vi "Raw Data.vi"(0 "reference in":refnum<class "Advantech.lvclass">, 5 "error in (no error)":errorcluster) -> (14 "reference out":refnum<class "Advantech.lvclass">, 15 "Raw Data":dbl, 19 "error out":errorcluster)   [LabVIEW 2013, in "Advantech.lvclass"]
uses:
  Advantech.lvclass
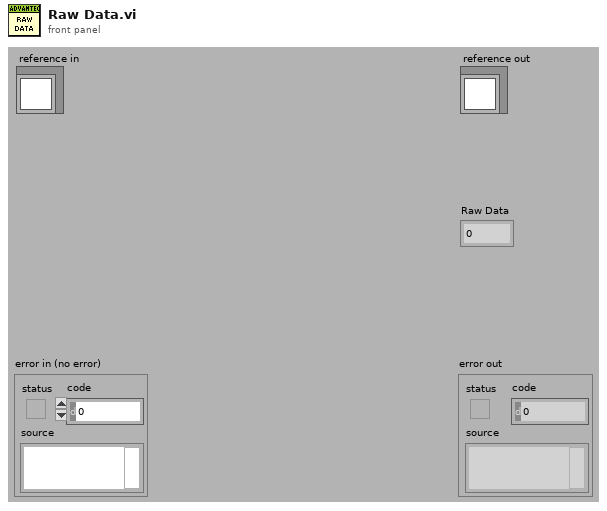
[diagram p1: front panel]
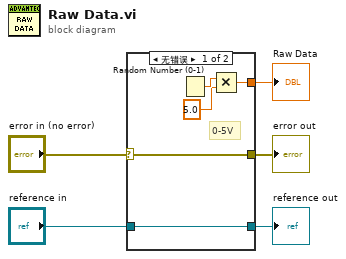
[diagram p0: block diagram]
diagram:
  n1 = case shown="无错误" "error in (no error)" {
    selector: "error in (no error)" -> [w9 w12]
    tunnel: [w9 w12] -> w4
    tunnel: [w10 w11] -> w2
    tunnel: "reference in" -> [w10 w11]
    tunnel: [w6 _] -> w1
    frame No Error {
      # "0-5V"
      n2 = Random Number (0-1)() -> (number: 0 to 1=w8:dbl)
      n3 = Multiply(x=w8, y=5.0) -> (x*y=w6:dbl)
    }
    frame Error {
    }
  }
  "error out" <- w4
  "reference out" <- w2
  "Raw Data" <- w1
